vi "RS232 通訊 KEYENCE ML-G9300.vi"(7 "Enum":T1(ring)=enum."雷射觸發", 8 "error in":errorcluster, 10 "命令字串":string="RE", 11 "VISA resource name":refnum<visa-resource-name>) -> (0 "error out":errorcluster, 2 "回復訊息":string, 3 "VISA resource name out":refnum<visa-resource-name>)   [LabVIEW 2013]
uses:
  <vilib>/Instr/_visa.llb/VISA Configure Serial Port (Instr).vi
panel:
  in  "Error Table":string[][](table)=[["雷射通訊初始化異常!"], ["雷射未準備就緒!"], ["雷射觸發失敗!"], ["雷射通訊關閉異常!"], ["雷射XY座標值讀"], ["雷射XY座標值寫入異常!"], ["請求雷射程式編號prog#異常!"], ["開起雷射導向光異常!"], ["關閉雷射導向光異常!"]]
  out "substring":string
  out "after substring":string
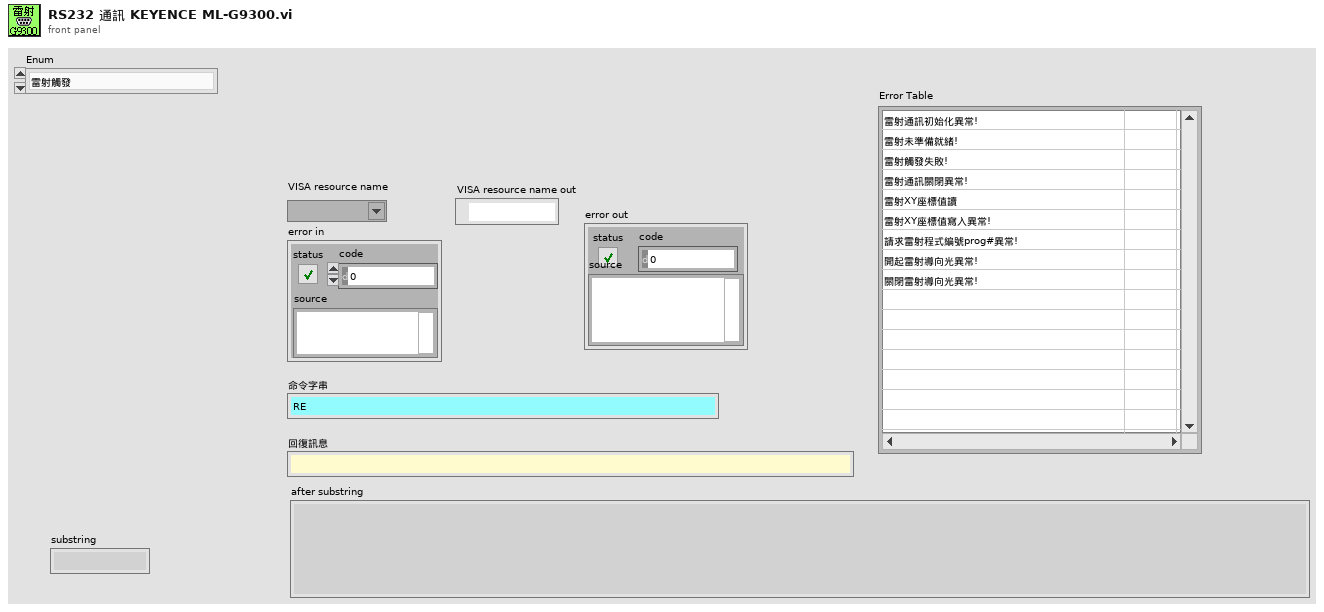
[diagram p1: front panel]
types:
  T1 = enum16{"RS232_Init ", "雷射準備訊號", "雷射觸發", "RS232_Close", "寫入雷射XY座標值與角度", "請求程式編號prog所有資訊", "開起導向光", "關閉導向光"}
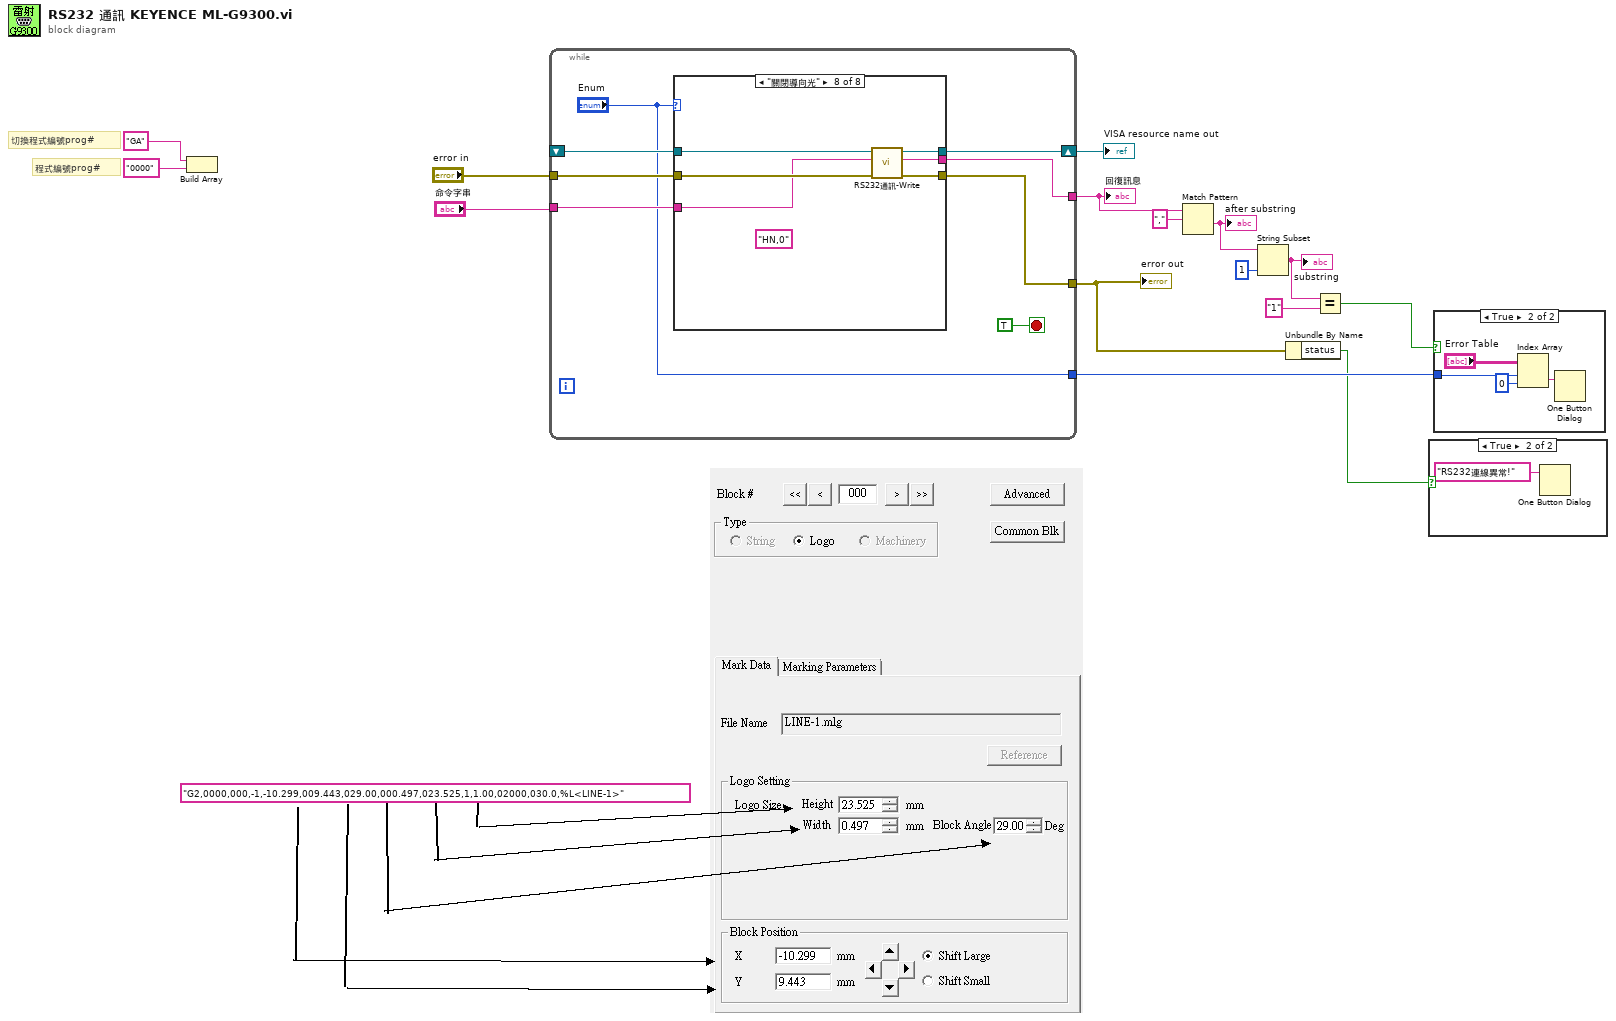
[diagram p0: block diagram]
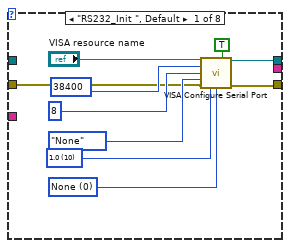
[diagram p4: hidden frame]
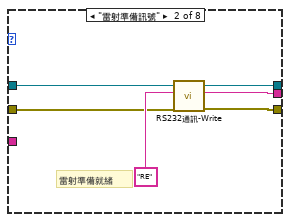
[diagram p5: hidden frame]
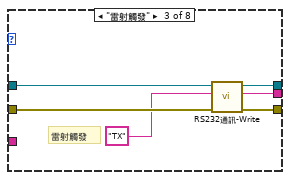
[diagram p6: hidden frame]
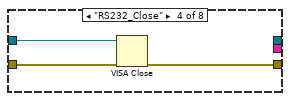
[diagram p7: hidden frame]
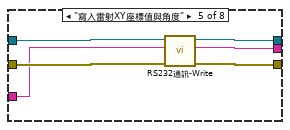
[diagram p8: hidden frame]
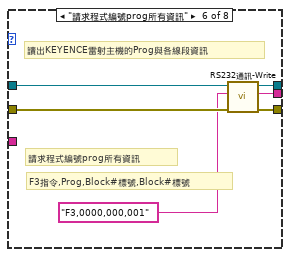
[diagram p9: hidden frame]
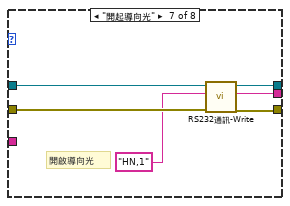
[diagram p10: hidden frame]
diagram:
  (unwired) "G2,0000,000,-1,-10.299,009.443,029.00,000.497,023.525,1,1.00,02000,030.0,%L<LINE-1>"
  # "程式編號prog#"
  # "切換程式編號prog#"
  n1 = Build Array("GA", "0000") -> ()  [unwired: 1 out]
  n2 = while {
    shift-right: [w19] -> w4
    shift-left: _ -> [w22]
    tunnel: [w18] -> w14
    tunnel: "error in" -> [w21]
    tunnel: [w17] -> w3
    tunnel: "命令字串" -> [w20]
    tunnel: ["Enum"] -> w8
    stop <- TRUE stop-if-true
    n3 = case shown="\"關閉導向光\"" "Enum" {
      tunnel: [w28 w36 w45 _ w54 w59 w65 w71] -> w19
      tunnel: w22 -> [_ w35 w40 w48 w53 w60 w66 w72]
      tunnel: w21 -> [w26 w34 w42 w46 w52 w56 w62 w68]
      tunnel: [w25 w37 w43 w47 w51 w57 w63 w69] -> w17
      tunnel: w20 -> [_ _ _ _ w49 _ _ w67]
      tunnel: [_ w39 w44 _ w50 w58 w64 w70] -> w18
      frame "RS232_Init ", Default {
        w33 = u16 0 items=["None", "XON/XOFF", "RTS/CTS", "XON/XOFF & RTS/CTS", "DTR/DSR", "XON/XOFF & DTR/DSR"] ("flow control (0:none)")
        w32 = u16 10 items=["1.0"=10, "1.5"=15, "2.0"=20] ("stop bits (10: 1 bit)")
        n4 = call-poly "VISA Configure Serial Port"("VISA resource name"="VISA resource name", "Enable Termination\nChar (T)"=TRUE ("Enable Termination\nChar (T)"), "baud rate (9600)"=u32 38400, "data bits (8)"=u16 8, "parity (0:none)"=enum16{"None", "Odd", "Even", "Mark", "Space"}."None", "error in (no error)"=w26, "stop bits (10: 1 bit)"=w32, "flow control (0:none)"=w33) -> ("VISA resource name out"=w28:refnum<visa-resource-name>, "error out"=w25:errorcluster)  [unwired: 6 in]
      }
      frame "雷射準備訊號" {
        # "雷射準備就緒"
        n5 = call "RS232通訊-Write.vi"("error in (no error)"=w34, "string"="RE", "VISA Refnum in"=w35) -> ("error out"=w37:errorcluster, "read buffer"=w39:string, "VISA resource name out"=w36:refnum<visa-resource-name>)  [unwired: 6 in]
      }
      frame "雷射觸發" {
        # "雷射觸發"
        n6 = call "RS232通訊-Write.vi"("error in (no error)"=w42, "string"="TX", "VISA Refnum in"=w40) -> ("error out"=w43:errorcluster, "read buffer"=w44:string, "VISA resource name out"=w45:refnum<visa-resource-name>)  [unwired: 6 in]
      }
      frame "RS232_Close" {
        n7 = VISA Close(VISA resource name=w48, error in (no error)=w46) -> (error out=w47:errorcluster)
      }
      frame "寫入雷射XY座標值與角度" {
        n8 = call "RS232通訊-Write.vi"("error in (no error)"=w52, "string"=w49, "VISA Refnum in"=w53) -> ("error out"=w51:errorcluster, "read buffer"=w50:string, "VISA resource name out"=w54:refnum<visa-resource-name>)  [unwired: 6 in]
      }
      frame "請求程式編號prog所有資訊" {
        # "讀出KEYENCE雷射主機的Prog與各線段資訊"
        # "F3指令,Prog,Block#標號,Block#標號"
        # "請求程式編號prog所有資訊"
        n9 = call "RS232通訊-Write.vi"("error in (no error)"=w56, "string"="F3,0000,000,001", "VISA Refnum in"=w60) -> ("error out"=w57:errorcluster, "read buffer"=w58:string, "VISA resource name out"=w59:refnum<visa-resource-name>)  [unwired: 6 in]
      }
      frame "開起導向光" {
        # "開啟導向光"
        n10 = call "RS232通訊-Write.vi"("error in (no error)"=w62, "string"="HN,1", "VISA Refnum in"=w66) -> ("error out"=w63:errorcluster, "read buffer"=w64:string, "VISA resource name out"=w65:refnum<visa-resource-name>)  [unwired: 6 in]
      }
      frame "關閉導向光" {
        (unwired) "HN,0"
        n11 = call "RS232通訊-Write.vi"("error in (no error)"=w68, "string"=w67, "VISA Refnum in"=w72) -> ("error out"=w69:errorcluster, "read buffer"=w70:string, "VISA resource name out"=w71:refnum<visa-resource-name>)  [unwired: 6 in]
      }
    }
  }
  "回復訊息" <- w14
  "VISA resource name out" <- w4
  "error out" <- w3
  n12 = Match Pattern(string=w14, regular expression=",") -> (after substring=w12:string)  [unwired: 1 in, 3 out]
  "after substring" <- w12
  n13 = String Subset(string=w12, length (rest)=1 ("length (rest)")) -> (substring=w10:string)  [unwired: 1 in]
  "substring" <- w10
  n14 = Unbundle By Name(w3) -> ("status"=w1:bool)
  n15 = Equal?(x=w10, y="1") -> (x = y?=w2:bool)
  n16 = case shown="True" w1 {
    frame False {
    }
    frame True {
      n17 = One Button Dialog(message="RS232連線異常!") -> ()  [unwired: 1 in, 1 out]
    }
  }
  n18 = case shown="True" w2 {
    tunnel: w8 -> [_ w75]
    frame False {
    }
    frame True {
      n19 = Index Array(array="Error Table", index (row)=w75, index (col)=0 ("disabled index (col)")) -> (element=w76:string)
      n20 = One Button Dialog(message=w76) -> ()  [unwired: 1 in, 1 out]
    }
  }
